vi "Autonomous Independent.vi"() -> ()   [LabVIEW 2020]
doc: "This VI is called when autonomous begins, and will automatically be terminated when autonomous ends. You can carry out timed or sensor driven robot movement independently without needing to return to the caller."
uses:
  <vilib>/Rock Robotics/WPI/ThirdParty/REV Robotics/REVLib/Typedef/Spark MAX Sensor Type.ctl
  <vilib>/Rock Robotics/WPI/Solenoid/WPI_SolenoidValue.ctl
  <vilib>/Rock Robotics/WPI/Utilities/WPI_GetSetVariantRefNum.vi
  <vilib>/Rock Robotics/Network Tables/NT Read String.vi
  <vilib>/Rock Robotics/Network Tables/NT Write Numeric Array.vi
  <vilib>/Rock Robotics/Network Tables/NT Write Number.vi
  Robot Global Data.vi
  <vilib>/Rock Robotics/WPI/Solenoid/WPI_SolenoidSetEnum.vi
  <vilib>/Rock Robotics/WPI/RobotDrive/WPI_RobotDriveArcadeDrive_Standard(NoSaturation).vi
panel:
  out "Right Drive Encoder 2":dbl format="%#.3f"
  out "Sensor Position 2":dbl
  out "Timestamp 2":u32
  out "Sensor Position":dbl
  out "Timestamp":u32
  in  "error in 2":errorcluster
  out "Real Yaw":dbl
  out "Right Drive Encoder":dbl format="%#.3f"
  in  "error in":errorcluster
  # "Be sure to right-click and choose Data Operations>>Make Current Value default if you want to save the array values with the VI"
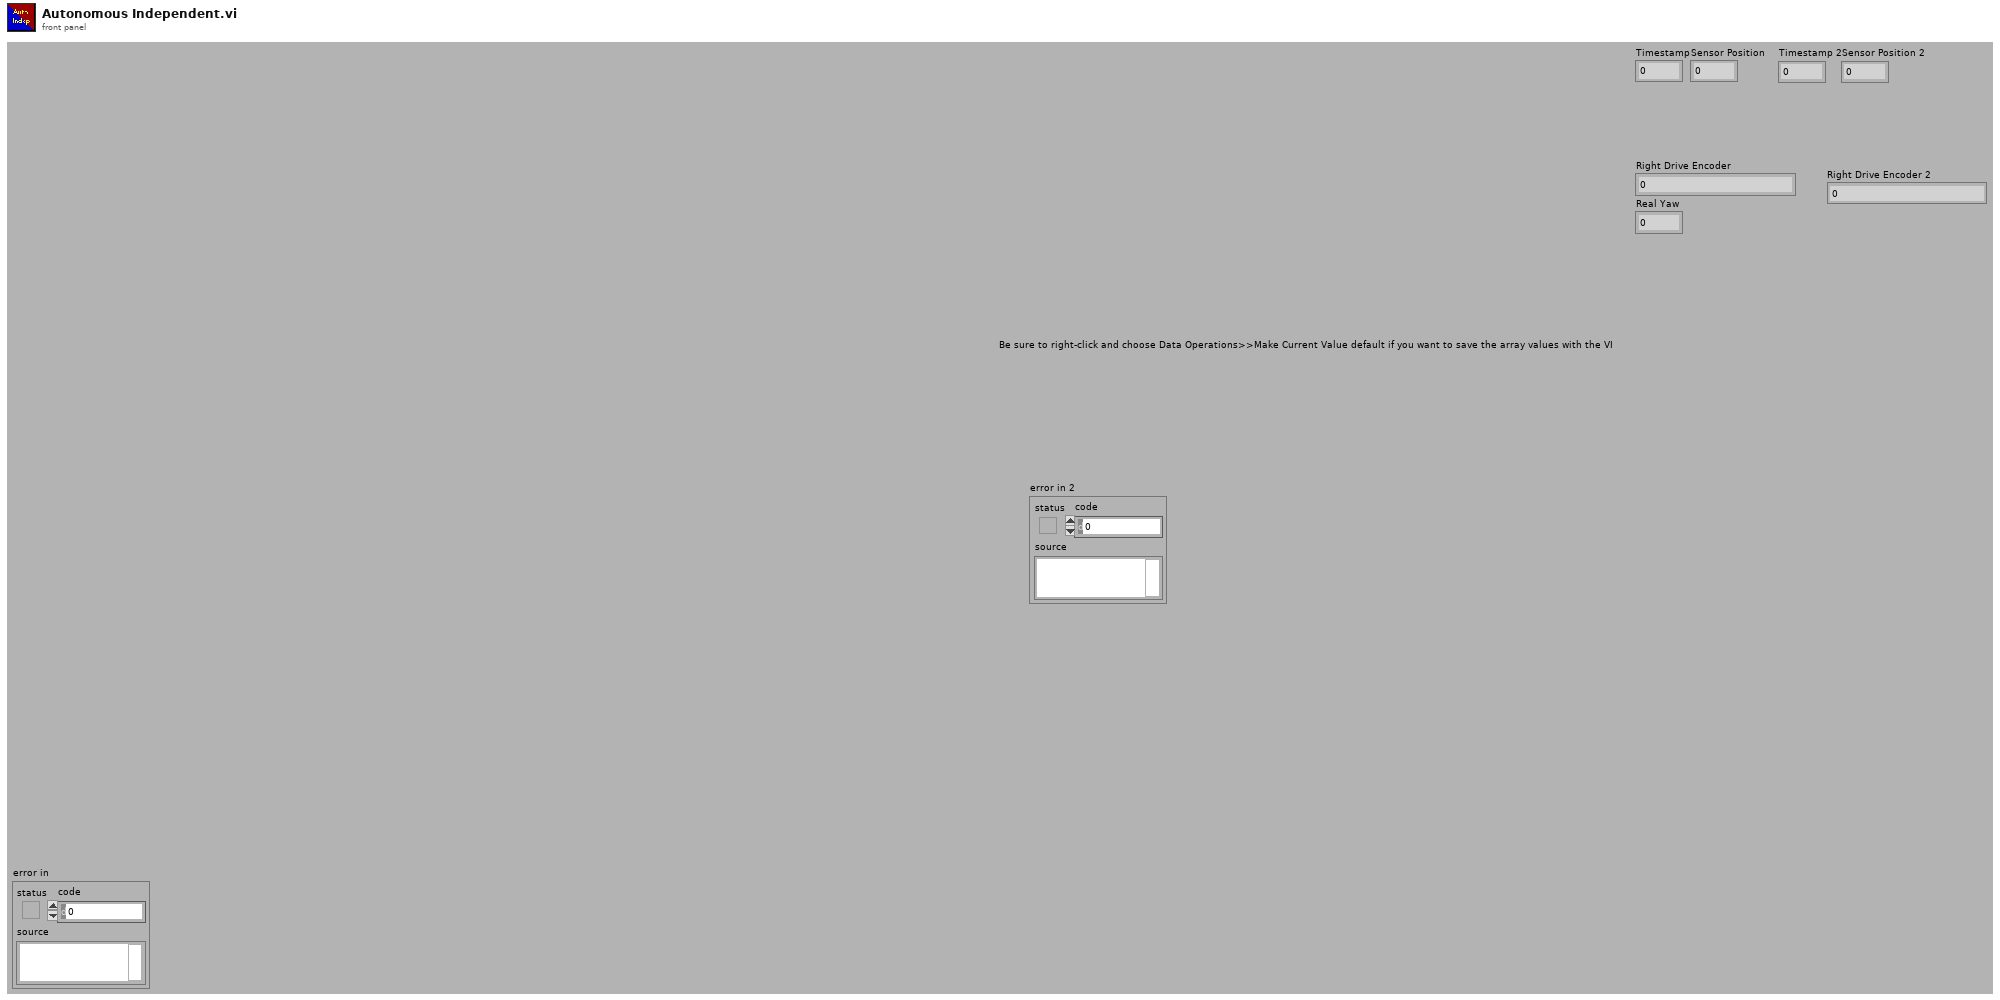
[diagram p1: front panel]
types:
  T1 = typedef "Spark MAX Sensor Type.ctl" = enum16{"No Sensor", "Hall Sensor", "Encoder", "-Not Available-", "Analog", "Alternate Encoder", "Duty Cycle"}
  T2 = typedef "WPI_JoystickDevRef.ctl" = cluster{"Device":T3}
  T3 = typedef "WPI_JoystickDeviceEnum.ctl" = enum16{"USB 0", "USB 1", "USB 2", "USB 3", "USB 4", "USB 5"}
  T4 = typedef "WPI_RobotDriveDevRef.ctl" = cluster{"DevStatus":errorcluster, "Motors[]":T5[], "Square Inputs":bool, "Max Output":dbl}
  T5 = typedef "WPI_MotorControlDeviceRef.ctl" = cluster{"DeviceStatus":errorcluster, "Type":T6, "PWM":cluster{"PWM Channel":T7, "DeadBand":T8}, "CAN":cluster{"Device Number":u8, "SetOutput VI Ref":variant, "GetOutput VI Ref":variant, "Enable VI Ref":variant, "Disable VI Ref":variant, "Data":variant}, "Invert":bool, "DIO PWM":cluster{"PWM \"Enable\" Channel":T7, "DIOChannel":T9, "PWM Rate":dbl}}
  T6 = typedef "WPI_MotorControlType.ctl" = enum16{"PWM", "CAN", "DIO PWM"}
  T7 = typedef "FPGA_DIOPWMChannel.ctl" = enum8{"PWM 0", "PWM 1", "PWM 2", "PWM 3", "PWM 4", "PWM 5", "PWM 6", "PWM 7", "PWM 8", "PWM 9", "PWM MXP 0", "PWM MXP 1", "PWM MXP 2", "PWM MXP 3", "PWM MXP 4", "PWM MXP 5", "PWM MXP 6", "PWM MXP 7", "PWM MXP 8", "PWM MXP 9", "Invalid"}
  T8 = typedef "WPI_PWMDeadband.ctl" = cluster{"Name":string, "maxPositivePwm":i32, "minPositivePwm":i32, "centerPwm":i32, "maxNegativePwm":i32, "minNegativePwm":i32, "angularRange":u16}
  T9 = typedef "FPGA_DIOChannel.ctl" = enum8{"DIO 0", "DIO 1", "DIO 2", "DIO 3", "DIO 4", "DIO 5", "DIO 6", "DIO 7", "DIO 8", "DIO 9", "DIO MXP 0", "DIO MXP 1", "DIO MXP 2", "DIO MXP 3", "DIO MXP 4", "DIO MXP 5", "DIO MXP 6", "DIO MXP 7", "DIO MXP 8", "DIO MXP 9", "DIO MXP 10", "DIO MXP 11", "DIO MXP 12", "DIO MXP 13", "DIO MXP 14", "DIO MXP 15", "SPI Port CS1", "SPI Port CS2", "SPI Port CS3", "SPI Port MISO", "SPI Port MOSI", "Invalid"}
  T10 = cluster{"Motors[][0]":T5, "Motors[][1]":T5, "Motors[][2]":T5, "Motors[][3]":T5, "Motors[][4]":T5, "Motors[][5]":T5, "Motors[][6]":T5, "Motors[][7]":T5, "Motors[][8]":T5}
  T11 = typedef "WPI_SolenoidValue.ctl" = enum16{"Off", "On", "Forward", "Reverse"}
  T12 = typedef "WPI_SolenoidDevRef.ctl" = cluster{"DevStatus":errorcluster, "Pneumatics Control Module":u8, "Forward Solenoid Channel":T13, "Reverse Solenoid Channel":T13}
  T13 = typedef "WPI_SolenoidChannel.ctl" = enum8{"Solenoid 0", "Solenoid 1", "Solenoid 2", "Solenoid 3", "Solenoid 4", "Solenoid 5", "Solenoid 6", "Solenoid 7", "Solenoid 8", "Solenoid 9", "Solenoid 10", "Solenoid 11", "Solenoid 12", "Solenoid 13", "Solenoid 14", "Solenoid 15", "Invalid"}
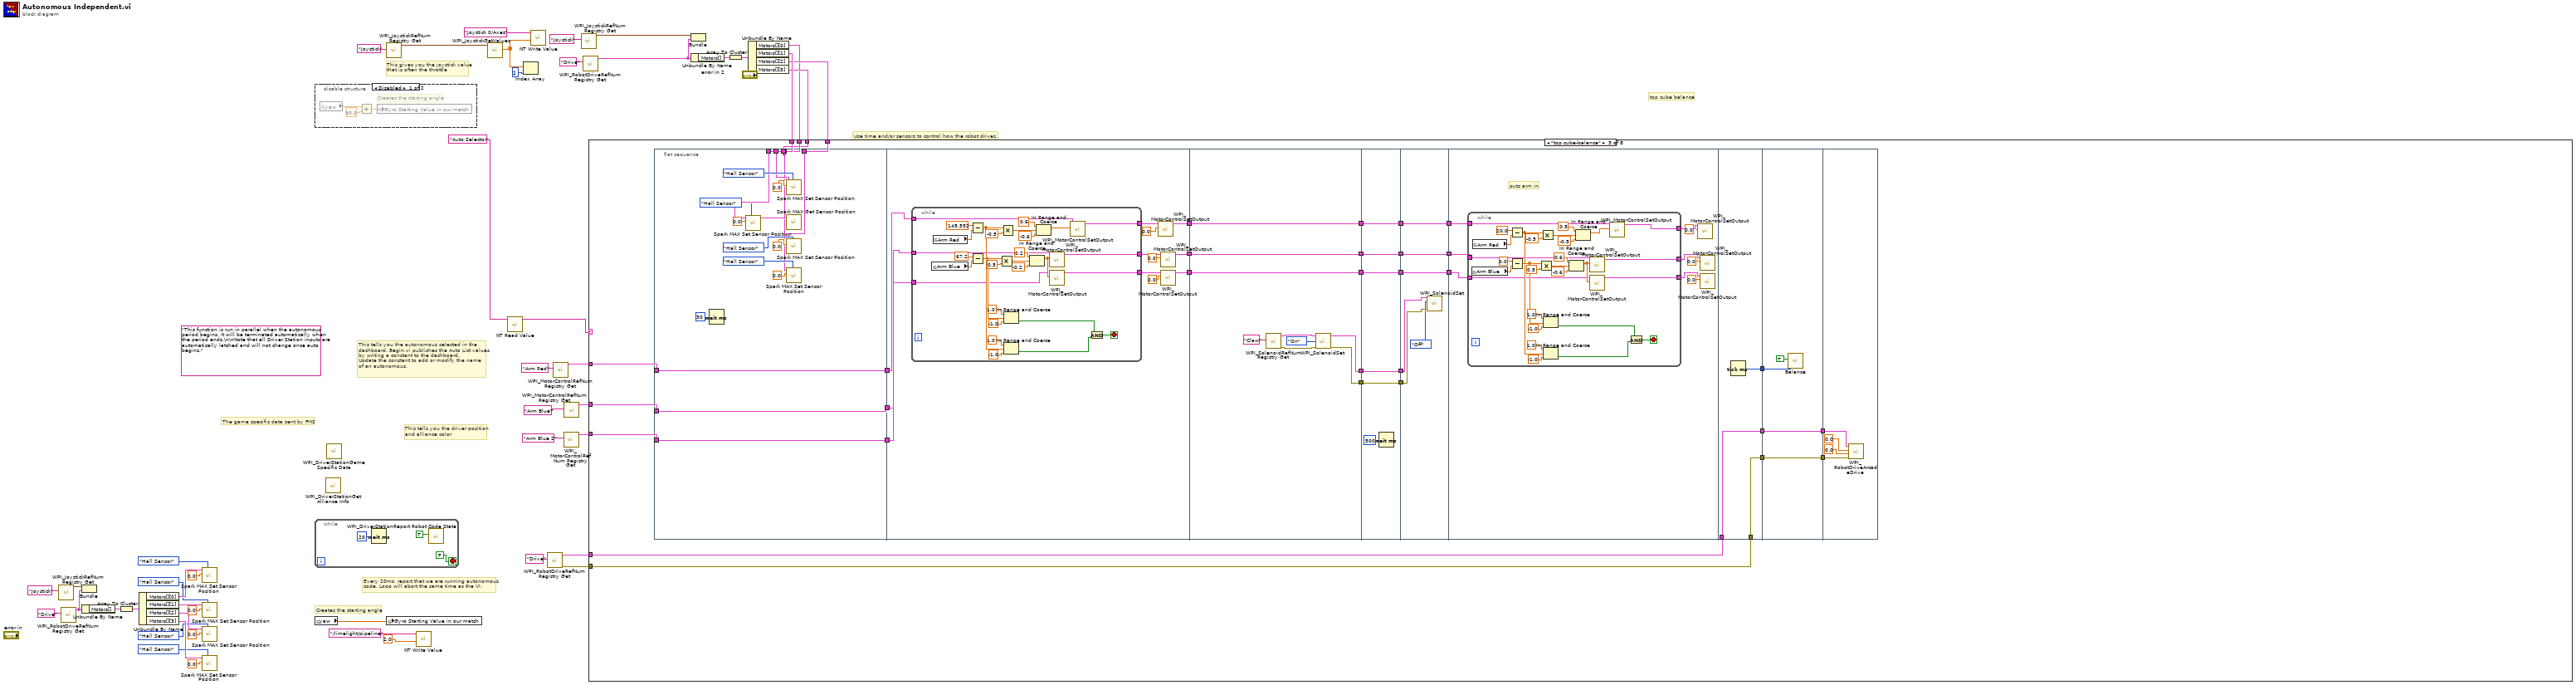
[diagram p0: block diagram]
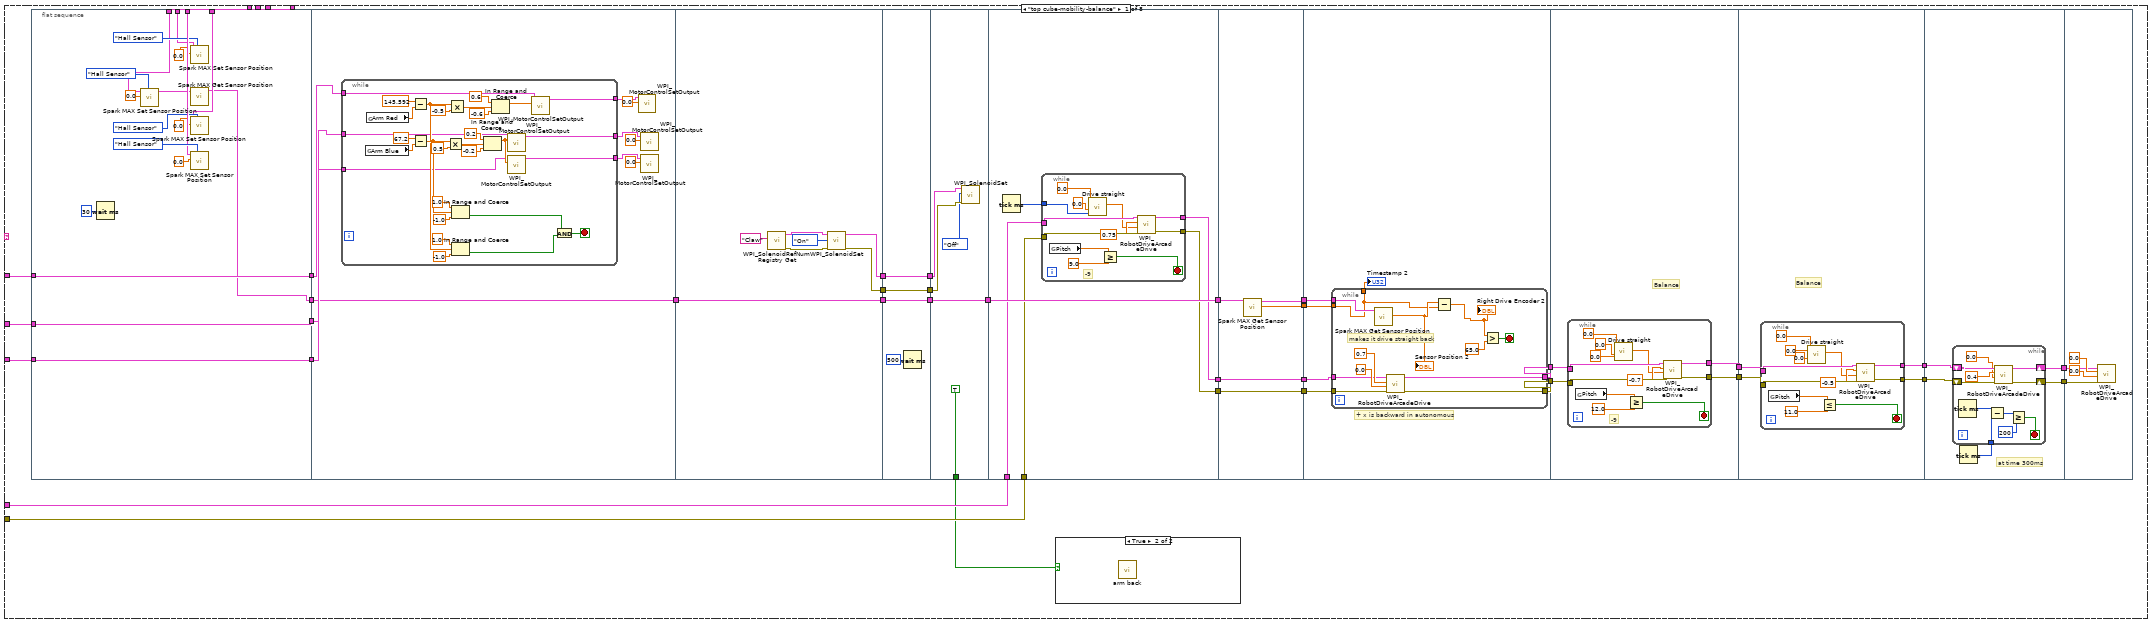
[diagram p3: hidden frame]
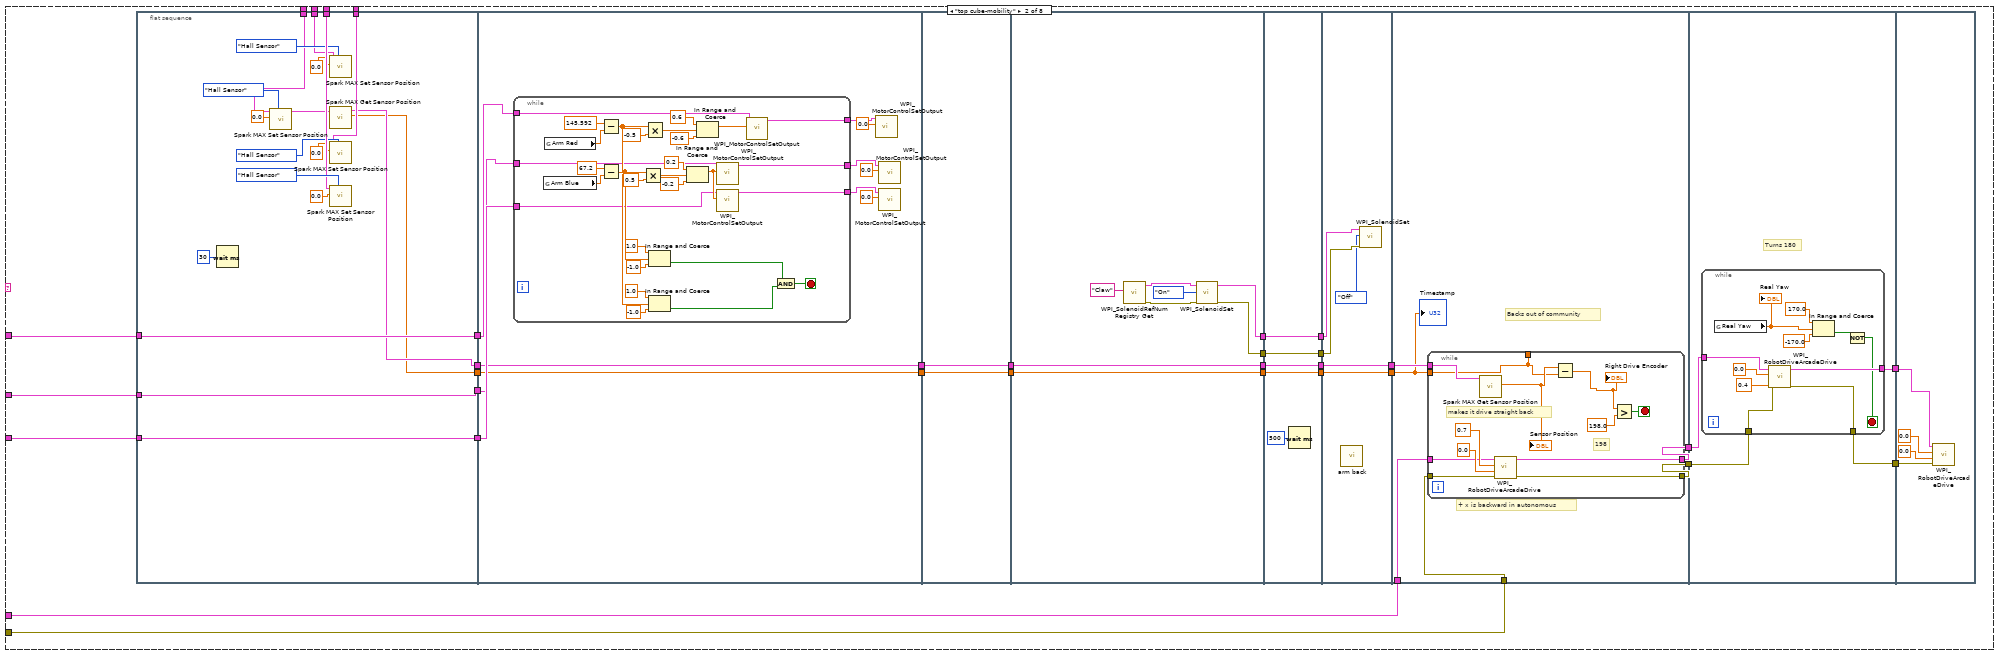
[diagram p5: hidden frame]
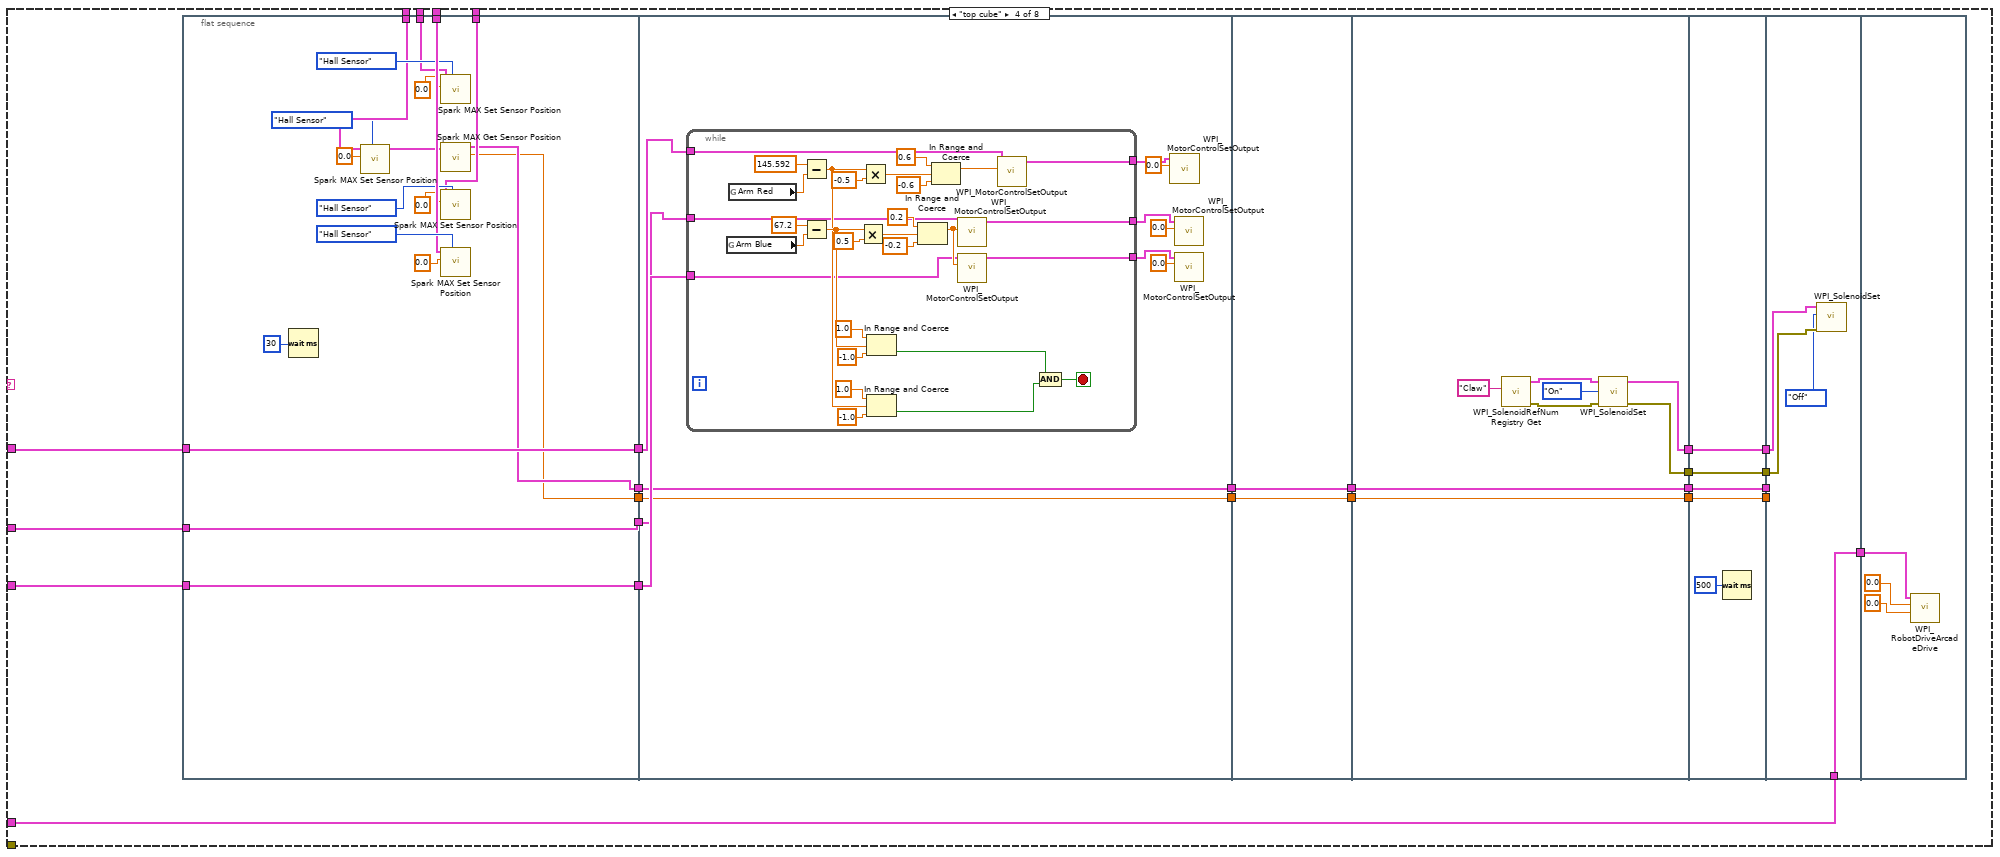
[diagram p6: hidden frame]
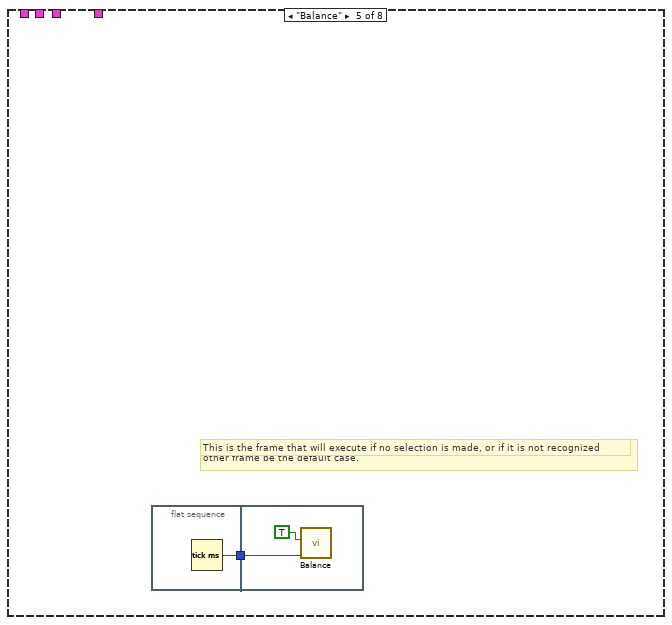
[diagram p7: hidden frame]
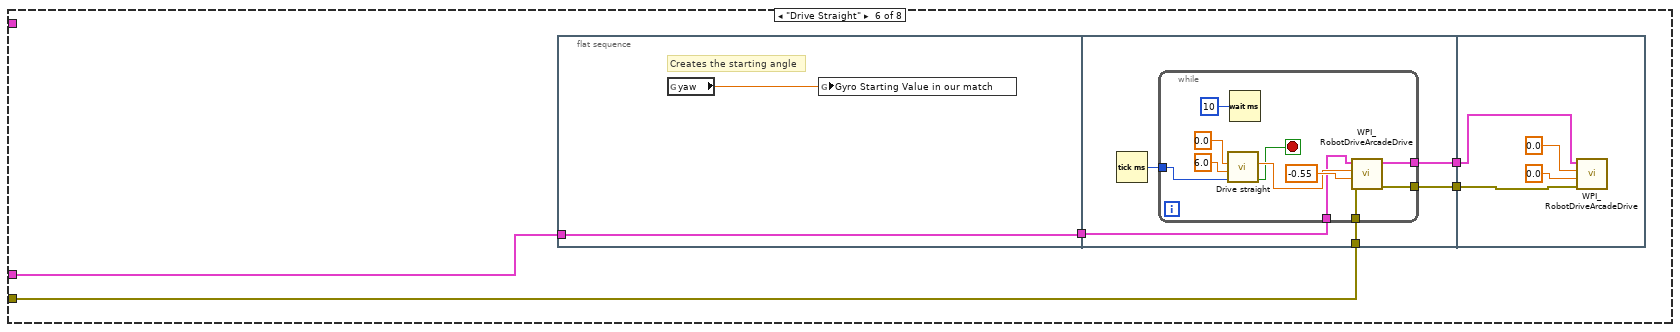
[diagram p8: hidden frame]
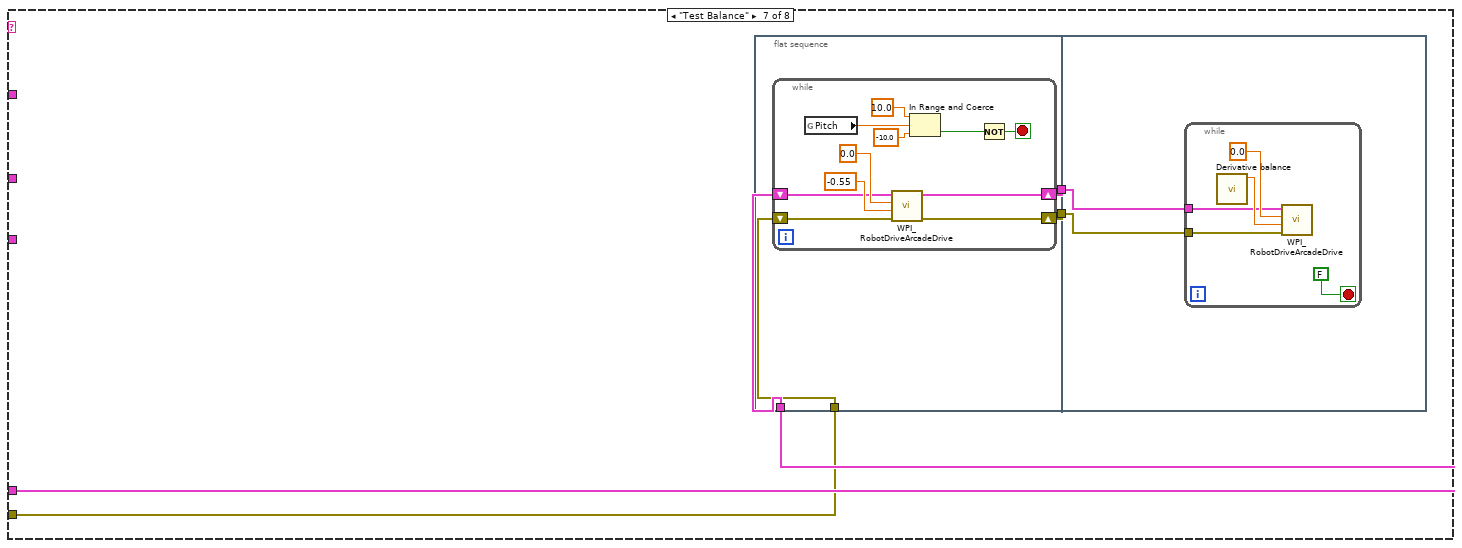
[diagram p9: hidden frame]
diagram:
  (unwired) "This function is run in parallel when the autonomous period begins. It will be terminated automatically when the period ends.\n\nNote that all Driver Station inputs are automatically latched and will not change once auto begins."
  # "top cube balance"
  # "Creates the starting angle"
  # "The game specific data sent by FMS"
  # "This tells you the autonomous selected in the \ndashboard. Begin.vi publishes the Auto List values\nby writing a constant to the dashboard.\nUpdate the constant to add or modify the name\nof an autonomous."
  # "Every 20ms, report that we are running autonomous\ncode. Loop will abort the same time as the VI."
  # "This gives you the joystick value\nthat is often the throttle"
  # "Use time and/or sensors to control how the robot drives."
  # "This tells you the driver position\nand alliance color"
  n1 = call <vilib>:"WPI_JoystickRefNum Registry Get.vi"("refnum name"="Joystick") -> ("JoystickDevRef"=w26:T2)  [unwired: 1 in, 9 out]
  n2 = call <vilib>:"WPI_RobotDriveRefNum Registry Get.vi"("refnum name"="Drive") -> ("RobotDriveDevRef"=w22:T4)  [unwired: 1 in, 9 out]
  n3 = Bundle("JoystickDevRef"=w26, "RobotDriveDevRef"=w22) -> ()  [unwired: 2 out]
  n4 = Unbundle By Name(w22) -> ("Motors[]"=w25:T5[])
  n5 = Array To Cluster(array=w25) -> (cluster=w24:T10)
  n6 = Unbundle By Name(w24) -> ("Motors[][0]"=w21:T5, "Motors[][1]"=w20:T5, "Motors[][2]"=w19:T5, "Motors[][3]"=w18:T5)
  n7 = call <vilib>:"Spark MAX Set Sensor Position.vi"("Sensor Type (Hall Sensor)"=Spark_MAX_Sensor_Type."Hall Sensor", "Position"=0.0, "MotorControlDeviceRef"=w21) -> ()  [unwired: 7 in, 2 out]
  n8 = call <vilib>:"Spark MAX Set Sensor Position.vi"("Sensor Type (Hall Sensor)"=Spark_MAX_Sensor_Type."Hall Sensor", "Position"=0.0, "MotorControlDeviceRef"=w20) -> ()  [unwired: 7 in, 2 out]
  n9 = call <vilib>:"Spark MAX Set Sensor Position.vi"("Sensor Type (Hall Sensor)"=Spark_MAX_Sensor_Type."Hall Sensor", "Position"=0.0, "MotorControlDeviceRef"=w19) -> ()  [unwired: 7 in, 2 out]
  n10 = call <vilib>:"Spark MAX Set Sensor Position.vi"("Sensor Type (Hall Sensor)"=Spark_MAX_Sensor_Type."Hall Sensor", "Position"=0.0, "MotorControlDeviceRef"=w18) -> ()  [unwired: 7 in, 2 out]
  n11 = disable-structure shown="Disabled" {
    frame Disabled {
      # "Creates the starting angle"
      n12 = global read "Robot Global Data.vi" "yaw"() -> (w49:dbl)
      n13 = Add(x=w49, y=90.0) -> (x+y=w50:dbl)
      n14 = global write "Robot Global Data.vi" "Gyro Starting Value in our match"(w50) -> ()
    }
    frame Enabled {
    }
  }
  n15 = while {
    stop <- FALSE stop-if-true
    n16 = Wait (ms)(milliseconds to wait=u32 20) -> ()  [unwired: 1 out]
    n17 = call <vilib>:"WPI_DriverStationReport Robot Code State.vi"("Autonomous"=TRUE) -> ()  [unwired: 10 in, 1 out]
  }
  n18 = global read "Robot Global Data.vi" "yaw"() -> (w40:dbl)
  n19 = call <vilib>:"WPI_DriverStationGet Alliance Info.vi"() -> ()  [unwired: 12 out]
  n20 = call <vilib>:"WPI_DriverStationGame Specific Data.vi"() -> ()  [unwired: 11 in, 1 out]
  n21 = call <vilib>:"WPI_JoystickRefNum Registry Get.vi"("refnum name"="Joystick") -> ("JoystickDevRef"=w46:T2)  [unwired: 1 in, 9 out]
  n22 = global write "Robot Global Data.vi" "Gyro Starting Value in our match"(w40) -> ()
  n23 = call-poly <vilib>:"NT Write Value.vi"("value"=2.0, "name"="/limelight/pipeline" ("Name")) -> ()  [unwired: 9 in, 1 out]
  n24 = call <vilib>:"WPI_JoystickGetValues.vi"("JoystickDevRef"=w46) -> ("Axes"=w42:dbl[])  [unwired: 6 in, 4 out]
  n25 = call-poly <vilib>:"NT Read Value.vi"("name"="Auto Selector" ("Name")) -> ("value"=w43:string)  [unwired: 8 in, 2 out]
  n26 = Index Array(array=w42, index=2) -> ()  [unwired: 1 out]
  n27 = call-poly <vilib>:"NT Write Value.vi"("value"=w42, "name"="Joystick 0/Axes" ("Name")) -> ()  [unwired: 9 in, 1 out]
  n28 = call <vilib>:"WPI_RobotDriveRefNum Registry Get.vi"("refnum name"="Drive") -> ("error out"=w29:errorcluster, "RobotDriveDevRef"=w30:T4)  [unwired: 9 in]
  n29 = call <vilib>:"WPI_MotorControlRefNum Registry Get.vi"("refnum name"="Arm Red") -> ("MotorControlDevRef"=w34:T5)  [unwired: 9 in, 1 out]
  n30 = call <vilib>:"WPI_MotorControlRefNum Registry Get.vi"("refnum name"="Arm Blue 2") -> ("MotorControlDevRef"=w32:T5)  [unwired: 9 in, 1 out]
  n31 = call <vilib>:"WPI_MotorControlRefNum Registry Get.vi"("refnum name"="Arm Blue") -> ("MotorControlDevRef"=w33:T5)  [unwired: 9 in, 1 out]
  n32 = call <vilib>:"WPI_JoystickRefNum Registry Get.vi"("refnum name"="Joystick") -> ("JoystickDevRef"=w7:T2)  [unwired: 1 in, 9 out]
  n33 = call <vilib>:"WPI_RobotDriveRefNum Registry Get.vi"("refnum name"="Drive") -> ("RobotDriveDevRef"=w10:T4)  [unwired: 1 in, 9 out]
  n34 = Bundle("JoystickDevRef"=w7, "RobotDriveDevRef"=w10) -> ()  [unwired: 2 out]
  n35 = Unbundle By Name(w10) -> ("Motors[]"=w8:T5[])
  n36 = Array To Cluster(array=w8) -> (cluster=w9:T10)
  n37 = Unbundle By Name(w9) -> ("Motors[][0]"=w1:T5, "Motors[][1]"=w4:T5, "Motors[][2]"=w2:T5, "Motors[][3]"=w3:T5)
  n38 = case shown="\"top cube-balance\"" w43 {
    tunnel: w34 -> [w90 w289 w431 w592 _ _ _ _]
    tunnel: w33 -> [w89 w288 w430 w591 _ _ _ _]
    tunnel: w32 -> [w88 w287 w429 w590 _ _ _ _]
    tunnel: w30 -> [w72 w282 w428 w567 _ w679 w708 _]
    tunnel: w29 -> [w71 w281 w427 _ _ w678 w707 _]
    tunnel: w4 -> [w77 w267 w425 w577 _ _ _ _]
    tunnel: w3 -> [w76 w266 w423 w576 _ _ _ _]
    tunnel: w2 -> [w75 w265 w422 w575 _ _ _ _]
    tunnel: w1 -> [w74 w264 w424 w574 _ _ _ _]
    frame "top cube-mobility-balance" {
      n39 = flat-sequence {
        tunnel: w88 -> [w108]
        tunnel: w89 -> [w107]
        tunnel: w90 -> [w106]
        tunnel: [w108] -> w83
        tunnel: [w96] -> w80
        tunnel: [w107] -> w79
        tunnel: [w106] -> w78
        tunnel: w77 -> [w94]
        tunnel: w76 -> [w103]
        tunnel: w75 -> [w100]
        tunnel: w74 -> [w97]
        tunnel: w83 -> [w118]
        tunnel: [w117] -> w55
        tunnel: w80 -> [w117]
        tunnel: w79 -> [w115]
        tunnel: w78 -> [w116]
        tunnel: [w154] -> w87
        tunnel: [w153] -> w85
        tunnel: [w152] -> w81
        tunnel: w55 -> [w152]
        tunnel: w87 -> [w158]
        tunnel: [w158] -> w86
        tunnel: w85 -> [w157]
        tunnel: [w157] -> w84
        tunnel: [w156] -> w82
        tunnel: w81 -> [w156]
        tunnel: w86 -> [w163]
        tunnel: w84 -> [w162]
        tunnel: [w161] -> w73
        tunnel: w82 -> [w161]
        tunnel: [TRUE] -> w54
        tunnel: w73 -> [w169]
        tunnel: [w169] -> w68
        tunnel: w72 -> [w167]
        tunnel: w71 -> [w166]
        tunnel: [w165] -> w66
        tunnel: [w164] -> w64
        tunnel: w68 -> [w184]
        tunnel: [w183] -> w67
        tunnel: w66 -> [w186]
        tunnel: [w186] -> w65
        tunnel: w64 -> [w185]
        tunnel: [w185] -> w63
        tunnel: [w182] -> w62
        tunnel: [w193] -> w70
        tunnel: [w192] -> w69
        tunnel: w67 -> [w191]
        tunnel: w65 -> [w190]
        tunnel: w63 -> [w189]
        tunnel: w62 -> [w188]
        tunnel: w70 -> [w209]
        tunnel: [w207] -> w61
        tunnel: w69 -> [w208]
        tunnel: [w206] -> w60
        tunnel: w61 -> [w225]
        tunnel: w60 -> [w224]
        tunnel: [w223] -> w59
        tunnel: [w222] -> w58
        tunnel: w59 -> [w241]
        tunnel: w58 -> [w240]
        tunnel: [w239] -> w57
        tunnel: [w238] -> w56
        tunnel: w57 -> [w255]
        tunnel: w56 -> [w254]
        frame #0 {
          n40 = Wait (ms)(milliseconds to wait=u32 30) -> ()  [unwired: 1 out]
          n41 = call <vilib>:"Spark MAX Set Sensor Position.vi"("Sensor Type (Hall Sensor)"=Spark_MAX_Sensor_Type."Hall Sensor", "Position"=0.0, "MotorControlDeviceRef"=w94) -> ("MotorControlDeviceRef"=w93:T5)  [unwired: 7 in, 1 out]
          n42 = call <vilib>:"Spark MAX Set Sensor Position.vi"("Sensor Type (Hall Sensor)"=Spark_MAX_Sensor_Type."Hall Sensor", "Position"=0.0, "MotorControlDeviceRef"=w97) -> ()  [unwired: 7 in, 2 out]
          n43 = call <vilib>:"Spark MAX Get Sensor Position.vi"("MotorControlDevRef in"=w93) -> ("MotorControlDevRef out"=w96:T5)  [unwired: 7 in, 3 out]
          n44 = call <vilib>:"Spark MAX Set Sensor Position.vi"("Sensor Type (Hall Sensor)"=Spark_MAX_Sensor_Type."Hall Sensor", "Position"=0.0, "MotorControlDeviceRef"=w100) -> ()  [unwired: 7 in, 2 out]
          n45 = call <vilib>:"Spark MAX Set Sensor Position.vi"("Sensor Type (Hall Sensor)"=Spark_MAX_Sensor_Type."Hall Sensor", "Position"=0.0, "MotorControlDeviceRef"=w103) -> ()  [unwired: 7 in, 2 out]
        }
        frame #1 {
          n46 = while {
            tunnel: w116 -> [w124]
            tunnel: w115 -> [w123]
            tunnel: w118 -> [w122]
            tunnel: [w119] -> w114
            tunnel: [w121] -> w113
            tunnel: [w120] -> w112
            stop <- w147 stop-if-true
            n47 = global read "Robot Global Data.vi" "Arm Blue"() -> (w127:dbl)
            n48 = global read "Robot Global Data.vi" "Arm Red"() -> (w138:dbl)
            n49 = Subtract(x=145.592, y=w138) -> (x-y=w125:dbl)
            n50 = Subtract(x=67.2, y=w127) -> (x-y=w126:dbl)
            n51 = Multiply(x=w126, y=0.5) -> (x*y=w135:dbl)
            n52 = Multiply(x=w125, y=-0.5) -> (x*y=w134:dbl)
            n53 = In Range and Coerce(upper limit=1.0, x=w126, lower limit=-1.0) -> (In Range?=w146:bool)  [unwired: 1 out]
            n54 = In Range and Coerce(upper limit=1.0, x=w125, lower limit=-1.0) -> (In Range?=w145:bool)  [unwired: 1 out]
            n55 = In Range and Coerce(upper limit=0.2, x=w135, lower limit=-0.2) -> (coerced(x)=w130:dbl)  [unwired: 1 out]
            n56 = In Range and Coerce(upper limit=0.6, x=w134, lower limit=-0.6) -> (coerced(x)=w131:dbl)  [unwired: 1 out]
            n57 = call <vilib>:"WPI_MotorControlSetOutput.vi"("Output"=w130, "MotorControlDevRef"=w123) -> ("MotorControlDevRef"=w119:T5)  [unwired: 7 in, 2 out]
            n58 = call <vilib>:"WPI_MotorControlSetOutput.vi"("Output"=w130, "MotorControlDevRef"=w122) -> ("MotorControlDevRef"=w121:T5)  [unwired: 7 in, 2 out]
            n59 = call <vilib>:"WPI_MotorControlSetOutput.vi"("Output"=w131, "MotorControlDevRef"=w124) -> ("MotorControlDevRef"=w120:T5)  [unwired: 7 in, 2 out]
            n60 = And(x=w146, y=w145) -> (x .and. y?=w147:bool)
          }
          n61 = call <vilib>:"WPI_MotorControlSetOutput.vi"("Output"=0.0, "MotorControlDevRef"=w112) -> ()  [unwired: 7 in, 3 out]
          n62 = call <vilib>:"WPI_MotorControlSetOutput.vi"("Output"=0.0, "MotorControlDevRef"=w114) -> ()  [unwired: 7 in, 3 out]
          n63 = call <vilib>:"WPI_MotorControlSetOutput.vi"("Output"=0.0, "MotorControlDevRef"=w113) -> ()  [unwired: 7 in, 3 out]
        }
        frame #2 {
          n64 = call <vilib>:"WPI_SolenoidRefNum Registry Get.vi"("refnum name"="Claw") -> ("error out"=w151:errorcluster, "SolenoidDevRef"=w150:T12)  [unwired: 9 in]
          n65 = call-poly <vilib>:"WPI_SolenoidSet.vi"("error in (no error)"=w151, "Value"=WPI_SolenoidValue."On", "SolenoidDevRef"=w150) -> ("error out"=w153:errorcluster, "SolenoidDevRef"=w154:T12)  [unwired: 7 in]
        }
        frame #3 {
          n66 = Wait (ms)(milliseconds to wait=u32 500) -> ()  [unwired: 1 out]
        }
        frame #4 {
          n67 = call-poly <vilib>:"WPI_SolenoidSet.vi"("error in (no error)"=w162, "Value"=WPI_SolenoidValue."Off", "SolenoidDevRef"=w163) -> ()  [unwired: 7 in, 2 out]
        }
        frame #5 {
          n68 = Tick Count (ms)() -> (millisecond timer value=w168:u32)
          n69 = while {
            tunnel: [w179] -> w165
            tunnel: w167 -> [w178]
            tunnel: w166 -> [w177]
            tunnel: [w175] -> w164
            tunnel: w168 -> [w171]
            stop <- w181 stop-if-true
            # "-9"
            n70 = global read "Robot Global Data.vi" "Pitch"() -> (w176:dbl)
            n71 = call "Drive straight.vi"("Start Time"=w171, "Length(seconds)"=0.0, "Desired angle"=0.0) -> ("X Power"=w172:dbl)  [unwired: 7 in, 1 out]
            n72 = Greater Or Equal?(x=w176, y=9.0) -> (x >= y?=w181:bool)
            n73 = call-poly <vilib>:"WPI_RobotDriveArcadeDrive.vi"("error in (no error)"=w177, "Y axis value"=w172, "X axis value"=0.75 ("Y axis value"), "RobotDriveDevRef"=w178) -> ("error out"=w175:errorcluster, "RobotDriveDevRef"=w179:T4)  [unwired: 5 in, 1 out]
          }
        }
        frame #6 {
          n74 = call <vilib>:"Spark MAX Get Sensor Position.vi"("MotorControlDevRef in"=w184) -> ("Sensor Position"=w182:dbl, "MotorControlDevRef out"=w183:T5)  [unwired: 7 in, 2 out]
        }
        frame #7 {
          # "+ x is backward in autonomous"
          n75 = while {
            tunnel: [w203] -> w193
            tunnel: [w202] -> w192
            tunnel: w190 -> [w200]
            tunnel: w191 -> [w198]
            tunnel: w189 -> [w195]
            tunnel: w188 -> [w194]
            tunnel: [w194] -> w187
            stop <- w201 stop-if-true
            # "makes it drive straight back"
            n76 = call <vilib>:"Spark MAX Get Sensor Position.vi"("MotorControlDevRef in"=w198) -> ("Sensor Position"=w196:dbl)  [unwired: 7 in, 3 out]
            "Sensor Position 2" <- w196
            n77 = call-poly <vilib>:"WPI_RobotDriveArcadeDrive.vi"("error in (no error)"=w195, "Y axis value"=0.0, "X axis value"=0.7, "RobotDriveDevRef"=w200) -> ("error out"=w202:errorcluster, "RobotDriveDevRef"=w203:T4)  [unwired: 5 in, 1 out]
            n78 = Subtract(x=w196, y=w194) -> (x-y=w197:dbl)
            "Right Drive Encoder 2" <- w197
            n79 = Greater?(x=w197, y=65.0) -> (0:w201:bool)
          }
          "Timestamp 2" <- w187
        }
        frame #8 {
          # "Balance"
          n80 = while {
            tunnel: [w219] -> w207
            tunnel: w209 -> [w218]
            tunnel: w208 -> [w217]
            tunnel: [w215] -> w206
            stop <- w221 stop-if-true
            # "-9"
            n81 = global read "Robot Global Data.vi" "Pitch"() -> (w216:dbl)
            n82 = call "Drive straight.vi"("Start Time"=0.0, "Length(seconds)"=0.0, "Desired angle"=0.0) -> ("X Power"=w212:dbl)  [unwired: 7 in, 1 out]
            n83 = Greater Or Equal?(x=w216, y=12.0) -> (x >= y?=w221:bool)
            n84 = call-poly <vilib>:"WPI_RobotDriveArcadeDrive.vi"("error in (no error)"=w217, "Y axis value"=w212, "X axis value"=-0.7 ("Y axis value"), "RobotDriveDevRef"=w218) -> ("error out"=w215:errorcluster, "RobotDriveDevRef"=w219:T4)  [unwired: 5 in, 1 out]
          }
        }
        frame #9 {
          # "Balance"
          n85 = while {
            tunnel: [w235] -> w223
            tunnel: w225 -> [w234]
            tunnel: w224 -> [w233]
            tunnel: [w231] -> w222
            stop <- w237 stop-if-true
            n86 = global read "Robot Global Data.vi" "Pitch"() -> (w232:dbl)
            n87 = call "Drive straight.vi"("Start Time"=0.0, "Length(seconds)"=0.0, "Desired angle"=0.0) -> ("X Power"=w227:dbl)  [unwired: 7 in, 1 out]
            n88 = Less Or Equal?(x=w232, y=11.0) -> (x <= y?=w237:bool)
            n89 = call-poly <vilib>:"WPI_RobotDriveArcadeDrive.vi"("error in (no error)"=w233, "Y axis value"=w227, "X axis value"=-0.5 ("Y axis value"), "RobotDriveDevRef"=w234) -> ("error out"=w231:errorcluster, "RobotDriveDevRef"=w235:T4)  [unwired: 5 in, 1 out]
          }
        }
        frame #10 {
          # "at time 300ms"
          n90 = Tick Count (ms)() -> (millisecond timer value=w242:u32)
          n91 = while {
            shift-right: [w251] -> w239
            shift-left: w241 -> [w253]
            shift-right: [w250] -> w238
            shift-left: w240 -> [w252]
            tunnel: w242 -> [w248]
            stop <- w245 stop-if-true
            n92 = Tick Count (ms)() -> (millisecond timer value=w249:u32)
            n93 = Subtract(x=w249, y=w248) -> (x-y=w247:u32)
            n94 = call-poly <vilib>:"WPI_RobotDriveArcadeDrive.vi"("error in (no error)"=w252, "Y axis value"=0.0 ("X axis value"), "X axis value"=0.4 ("Y axis value"), "RobotDriveDevRef"=w253) -> ("error out"=w250:errorcluster, "RobotDriveDevRef"=w251:T4)  [unwired: 5 in, 1 out]
            n95 = Greater Or Equal?(x=w247, y=u32 200) -> (x >= y?=w245:bool)
          }
        }
        frame #11 {
          n96 = call-poly <vilib>:"WPI_RobotDriveArcadeDrive.vi"("error in (no error)"=w254, "Y axis value"=0.0, "X axis value"=0.0, "RobotDriveDevRef"=w255) -> ()  [unwired: 5 in, 3 out]
        }
      }
      n97 = case shown="True" w54 {
        frame False {
        }
        frame True {
          n98 = call "arm back.vi"() -> ()  [unwired: 12 in]
        }
      }
    }
    frame "top cube-mobility" {
      n99 = flat-sequence {
        tunnel: w287 -> [w308]
        tunnel: w288 -> [w307]
        tunnel: w289 -> [w306]
        tunnel: [w308] -> w276
        tunnel: [w296] -> w270
        tunnel: [w307] -> w269
        tunnel: [w306] -> w268
        tunnel: w267 -> [w293]
        tunnel: w266 -> [w303]
        tunnel: w265 -> [w300]
        tunnel: w264 -> [w297]
        tunnel: [w295] -> w258
        tunnel: w276 -> [w319]
        tunnel: [w318] -> w271
        tunnel: w270 -> [w318]
        tunnel: w269 -> [w316]
        tunnel: w268 -> [w317]
        tunnel: [w315] -> w259
        tunnel: w258 -> [w315]
        tunnel: [w350] -> w272
        tunnel: w271 -> [w350]
        tunnel: [w349] -> w260
        tunnel: w259 -> [w349]
        tunnel: [w358] -> w286
        tunnel: [w357] -> w284
        tunnel: [w356] -> w273
        tunnel: w272 -> [w356]
        tunnel: [w355] -> w261
        tunnel: w260 -> [w355]
        tunnel: w286 -> [w363]
        tunnel: [w363] -> w285
        tunnel: w284 -> [w362]
        tunnel: [w362] -> w283
        tunnel: [w361] -> w274
        tunnel: w273 -> [w361]
        tunnel: [w360] -> w262
        tunnel: w261 -> [w360]
        tunnel: w285 -> [w368]
        tunnel: w283 -> [w367]
        tunnel: [w366] -> w275
        tunnel: w274 -> [w366]
        tunnel: [w365] -> w263
        tunnel: w262 -> [w365]
        tunnel: [w374] -> w280
        tunnel: [w373] -> w279
        tunnel: w282 -> [w372]
        tunnel: w281 -> [w371]
        tunnel: w275 -> [w370]
        tunnel: w263 -> [w369]
        tunnel: w280 -> [w390]
        tunnel: w279 -> [w389]
        tunnel: [w388] -> w278
        tunnel: [w387] -> w277
        tunnel: w278 -> [w403]
        tunnel: w277 -> [w402]
        frame #0 {
          n100 = Wait (ms)(milliseconds to wait=u32 30) -> ()  [unwired: 1 out]
          n101 = call <vilib>:"Spark MAX Set Sensor Position.vi"("Sensor Type (Hall Sensor)"=Spark_MAX_Sensor_Type."Hall Sensor", "Position"=0.0, "MotorControlDeviceRef"=w293) -> ("MotorControlDeviceRef"=w292:T5)  [unwired: 7 in, 1 out]
          n102 = call <vilib>:"Spark MAX Set Sensor Position.vi"("Sensor Type (Hall Sensor)"=Spark_MAX_Sensor_Type."Hall Sensor", "Position"=0.0, "MotorControlDeviceRef"=w297) -> ()  [unwired: 7 in, 2 out]
          n103 = call <vilib>:"Spark MAX Get Sensor Position.vi"("MotorControlDevRef in"=w292) -> ("Sensor Position"=w295:dbl, "MotorControlDevRef out"=w296:T5)  [unwired: 7 in, 2 out]
          n104 = call <vilib>:"Spark MAX Set Sensor Position.vi"("Sensor Type (Hall Sensor)"=Spark_MAX_Sensor_Type."Hall Sensor", "Position"=0.0, "MotorControlDeviceRef"=w300) -> ()  [unwired: 7 in, 2 out]
          n105 = call <vilib>:"Spark MAX Set Sensor Position.vi"("Sensor Type (Hall Sensor)"=Spark_MAX_Sensor_Type."Hall Sensor", "Position"=0.0, "MotorControlDeviceRef"=w303) -> ()  [unwired: 7 in, 2 out]
        }
        frame #1 {
          n106 = while {
            tunnel: w317 -> [w325]
            tunnel: w316 -> [w324]
            tunnel: w319 -> [w323]
            tunnel: [w320] -> w314
            tunnel: [w322] -> w313
            tunnel: [w321] -> w312
            stop <- w348 stop-if-true
            n107 = global read "Robot Global Data.vi" "Arm Blue"() -> (w328:dbl)
            n108 = global read "Robot Global Data.vi" "Arm Red"() -> (w339:dbl)
            n109 = Subtract(x=145.592, y=w339) -> (x-y=w326:dbl)
            n110 = Subtract(x=67.2, y=w328) -> (x-y=w327:dbl)
            n111 = Multiply(x=w327, y=0.5) -> (x*y=w336:dbl)
            n112 = Multiply(x=w326, y=-0.5) -> (x*y=w335:dbl)
            n113 = In Range and Coerce(upper limit=1.0, x=w327, lower limit=-1.0) -> (In Range?=w347:bool)  [unwired: 1 out]
            n114 = In Range and Coerce(upper limit=1.0, x=w326, lower limit=-1.0) -> (In Range?=w346:bool)  [unwired: 1 out]
            n115 = In Range and Coerce(upper limit=0.2, x=w336, lower limit=-0.2) -> (coerced(x)=w331:dbl)  [unwired: 1 out]
            n116 = In Range and Coerce(upper limit=0.6, x=w335, lower limit=-0.6) -> (coerced(x)=w332:dbl)  [unwired: 1 out]
            n117 = call <vilib>:"WPI_MotorControlSetOutput.vi"("Output"=w331, "MotorControlDevRef"=w324) -> ("MotorControlDevRef"=w320:T5)  [unwired: 7 in, 2 out]
            n118 = call <vilib>:"WPI_MotorControlSetOutput.vi"("Output"=w331, "MotorControlDevRef"=w323) -> ("MotorControlDevRef"=w322:T5)  [unwired: 7 in, 2 out]
            n119 = call <vilib>:"WPI_MotorControlSetOutput.vi"("Output"=w332, "MotorControlDevRef"=w325) -> ("MotorControlDevRef"=w321:T5)  [unwired: 7 in, 2 out]
            n120 = And(x=w347, y=w346) -> (x .and. y?=w348:bool)
          }
          n121 = call <vilib>:"WPI_MotorControlSetOutput.vi"("Output"=0.0, "MotorControlDevRef"=w312) -> ()  [unwired: 7 in, 3 out]
          n122 = call <vilib>:"WPI_MotorControlSetOutput.vi"("Output"=0.0, "MotorControlDevRef"=w314) -> ()  [unwired: 7 in, 3 out]
          n123 = call <vilib>:"WPI_MotorControlSetOutput.vi"("Output"=0.0, "MotorControlDevRef"=w313) -> ()  [unwired: 7 in, 3 out]
        }
        frame #2 {
        }
        frame #3 {
          n124 = call <vilib>:"WPI_SolenoidRefNum Registry Get.vi"("refnum name"="Claw") -> ("error out"=w354:errorcluster, "SolenoidDevRef"=w353:T12)  [unwired: 9 in]
          n125 = call-poly <vilib>:"WPI_SolenoidSet.vi"("error in (no error)"=w354, "Value"=WPI_SolenoidValue."On", "SolenoidDevRef"=w353) -> ("error out"=w357:errorcluster, "SolenoidDevRef"=w358:T12)  [unwired: 7 in]
        }
        frame #4 {
          n126 = Wait (ms)(milliseconds to wait=u32 500) -> ()  [unwired: 1 out]
        }
        frame #5 {
          n127 = call "arm back.vi"() -> ()  [unwired: 12 in]
          n128 = call-poly <vilib>:"WPI_SolenoidSet.vi"("error in (no error)"=w367, "Value"=WPI_SolenoidValue."Off", "SolenoidDevRef"=w368) -> ()  [unwired: 7 in, 2 out]
        }
        frame #6 {
          # "Backs out of community"
          # "+ x is backward in autonomous"
          n129 = while {
            tunnel: [w384] -> w374
            tunnel: [w383] -> w373
            tunnel: w372 -> [w381]
            tunnel: w371 -> [w380]
            tunnel: w370 -> [w378]
            tunnel: w369 -> [w375]
            tunnel: [w375] -> _
            stop <- w382 stop-if-true
            # "198"
            # "makes it drive straight back"
            n130 = call <vilib>:"Spark MAX Get Sensor Position.vi"("MotorControlDevRef in"=w378) -> ("Sensor Position"=w376:dbl)  [unwired: 7 in, 3 out]
            "Sensor Position" <- w376
            n131 = call-poly <vilib>:"WPI_RobotDriveArcadeDrive.vi"("error in (no error)"=w380, "Y axis value"=0.0, "X axis value"=0.7, "RobotDriveDevRef"=w381) -> ("error out"=w383:errorcluster, "RobotDriveDevRef"=w384:T4)  [unwired: 5 in, 1 out]
            n132 = Subtract(x=w376, y=w375) -> (x-y=w377:dbl)
            "Right Drive Encoder" <- w377
            n133 = Greater?(x=w377, y=198.0) -> (0:w382:bool)
          }
          "Timestamp" <- w369
        }
        frame #7 {
          # "Turns 180"
          n134 = while {
            tunnel: w390 -> [w399]
            tunnel: w389 -> [w398]
            tunnel: [w397] -> w388
            tunnel: [w396] -> w387
            stop <- w391 stop-if-true
            n135 = global read "Robot Global Data.vi" "Real Yaw"() -> (w393:dbl)
            "Real Yaw" <- w393
            n136 = call-poly <vilib>:"WPI_RobotDriveArcadeDrive.vi"("error in (no error)"=w398, "Y axis value"=0.4, "X axis value"=0.0, "RobotDriveDevRef"=w399) -> ("error out"=w396:errorcluster, "RobotDriveDevRef"=w397:T4)  [unwired: 5 in, 1 out]
            n137 = In Range and Coerce(upper limit=170.0, x=w393, lower limit=-170.0) -> (In Range?=w392:bool)  [unwired: 1 out]
            n138 = Not(x=w392) -> (.not. x?=w391:bool)
          }
        }
        frame #8 {
          n139 = call-poly <vilib>:"WPI_RobotDriveArcadeDrive.vi"("error in (no error)"=w402, "Y axis value"=0.0, "X axis value"=0.0, "RobotDriveDevRef"=w403) -> ()  [unwired: 5 in, 3 out]
        }
      }
    }
    frame "top cube-balance" {
      n140 = flat-sequence {
        tunnel: w429 -> [w455]
        tunnel: w430 -> [w454]
        tunnel: w431 -> [w453]
        tunnel: [w455] -> w438
        tunnel: [w454] -> w437
        tunnel: [w453] -> w436
        tunnel: w425 -> [w443]
        tunnel: [w439] -> _
        tunnel: w422 -> [w448]
        tunnel: w424 -> [w445]
        tunnel: w423 -> [w439]
        tunnel: w438 -> [w467]
        tunnel: w437 -> [w465]
        tunnel: w436 -> [w466]
        tunnel: [w459] -> w414
        tunnel: [w458] -> w410
        tunnel: [w457] -> w406
        tunnel: [w505] -> w435
        tunnel: [w504] -> w434
        tunnel: [w499] -> w415
        tunnel: w414 -> [w499]
        tunnel: [w498] -> w411
        tunnel: w410 -> [w498]
        tunnel: [w497] -> w407
        tunnel: w406 -> [w497]
        tunnel: w435 -> [w511]
        tunnel: [w511] -> w433
        tunnel: w434 -> [w510]
        tunnel: [w510] -> w432
        tunnel: [w508] -> w416
        tunnel: w415 -> [w508]
        tunnel: [w507] -> w412
        tunnel: w411 -> [w507]
        tunnel: [w506] -> w408
        tunnel: w407 -> [w506]
        tunnel: w433 -> [w517]
        tunnel: w432 -> [w516]
        tunnel: [w514] -> w417
        tunnel: w416 -> [w514]
        tunnel: [w513] -> w413
        tunnel: w412 -> [w513]
        tunnel: [w512] -> w409
        tunnel: w408 -> [w512]
        tunnel: w417 -> [w526]
        tunnel: w413 -> [w525]
        tunnel: w409 -> [w524]
        tunnel: w428 -> [w557]
        tunnel: w427 -> [w556]
        tunnel: [w558] -> w426
        tunnel: [w557] -> w420
        tunnel: [w556] -> w418
        tunnel: w426 -> [w561]
        tunnel: [w560] -> w421
        tunnel: w420 -> [w560]
        tunnel: [w559] -> w419
        tunnel: w418 -> [w559]
        tunnel: w421 -> [w564]
        tunnel: w419 -> [w563]
        frame #0 {
          n141 = Wait (ms)(milliseconds to wait=u32 30) -> ()  [unwired: 1 out]
          n142 = call <vilib>:"Spark MAX Set Sensor Position.vi"("Sensor Type (Hall Sensor)"=Spark_MAX_Sensor_Type."Hall Sensor", "Position"=0.0, "MotorControlDeviceRef"=w443) -> ("MotorControlDeviceRef"=w442:T5)  [unwired: 7 in, 1 out]
          n143 = call <vilib>:"Spark MAX Set Sensor Position.vi"("Sensor Type (Hall Sensor)"=Spark_MAX_Sensor_Type."Hall Sensor", "Position"=0.0, "MotorControlDeviceRef"=w445) -> ()  [unwired: 7 in, 2 out]
          n144 = call <vilib>:"Spark MAX Get Sensor Position.vi"("MotorControlDevRef in"=w442) -> ()  [unwired: 7 in, 4 out]
          n145 = call <vilib>:"Spark MAX Set Sensor Position.vi"("Sensor Type (Hall Sensor)"=Spark_MAX_Sensor_Type."Hall Sensor", "Position"=0.0, "MotorControlDeviceRef"=w448) -> ()  [unwired: 7 in, 2 out]
          n146 = call <vilib>:"Spark MAX Set Sensor Position.vi"("Sensor Type (Hall Sensor)"=Spark_MAX_Sensor_Type."Hall Sensor", "Position"=0.0, "MotorControlDeviceRef"=w439) -> ()  [unwired: 7 in, 2 out]
        }
        frame #1 {
          n147 = while {
            tunnel: w466 -> [w473]
            tunnel: w465 -> [w472]
            tunnel: w467 -> [w471]
            tunnel: [w468] -> w456
            tunnel: [w470] -> w464
            tunnel: [w469] -> w463
            stop <- w496 stop-if-true
            n148 = global read "Robot Global Data.vi" "Arm Blue"() -> (w476:dbl)
            n149 = global read "Robot Global Data.vi" "Arm Red"() -> (w487:dbl)
            n150 = Subtract(x=145.592, y=w487) -> (x-y=w474:dbl)
            n151 = Subtract(x=67.2, y=w476) -> (x-y=w475:dbl)
            n152 = Multiply(x=w475, y=0.5) -> (x*y=w484:dbl)
            n153 = Multiply(x=w474, y=-0.5) -> (x*y=w483:dbl)
            n154 = In Range and Coerce(upper limit=1.0, x=w475, lower limit=-1.0) -> (In Range?=w495:bool)  [unwired: 1 out]
            n155 = In Range and Coerce(upper limit=1.0, x=w474, lower limit=-1.0) -> (In Range?=w494:bool)  [unwired: 1 out]
            n156 = In Range and Coerce(upper limit=0.2, x=w484, lower limit=-0.2) -> (coerced(x)=w479:dbl)  [unwired: 1 out]
            n157 = In Range and Coerce(upper limit=0.6, x=w483, lower limit=-0.6) -> (coerced(x)=w480:dbl)  [unwired: 1 out]
            n158 = call <vilib>:"WPI_MotorControlSetOutput.vi"("Output"=w479, "MotorControlDevRef"=w472) -> ("MotorControlDevRef"=w468:T5)  [unwired: 7 in, 2 out]
            n159 = call <vilib>:"WPI_MotorControlSetOutput.vi"("Output"=w479, "MotorControlDevRef"=w471) -> ("MotorControlDevRef"=w470:T5)  [unwired: 7 in, 2 out]
            n160 = call <vilib>:"WPI_MotorControlSetOutput.vi"("Output"=w480, "MotorControlDevRef"=w473) -> ("MotorControlDevRef"=w469:T5)  [unwired: 7 in, 2 out]
            n161 = And(x=w495, y=w494) -> (x .and. y?=w496:bool)
          }
          n162 = call <vilib>:"WPI_MotorControlSetOutput.vi"("Output"=0.0, "MotorControlDevRef"=w463) -> ("MotorControlDevRef"=w459:T5)  [unwired: 7 in, 2 out]
          n163 = call <vilib>:"WPI_MotorControlSetOutput.vi"("Output"=0.0, "MotorControlDevRef"=w456) -> ("MotorControlDevRef"=w458:T5)  [unwired: 7 in, 2 out]
          n164 = call <vilib>:"WPI_MotorControlSetOutput.vi"("Output"=0.0, "MotorControlDevRef"=w464) -> ("MotorControlDevRef"=w457:T5)  [unwired: 7 in, 2 out]
        }
        frame #2 {
          n165 = call <vilib>:"WPI_SolenoidRefNum Registry Get.vi"("refnum name"="Claw") -> ("error out"=w503:errorcluster, "SolenoidDevRef"=w502:T12)  [unwired: 9 in]
          n166 = call-poly <vilib>:"WPI_SolenoidSet.vi"("error in (no error)"=w503, "Value"=WPI_SolenoidValue."On", "SolenoidDevRef"=w502) -> ("error out"=w504:errorcluster, "SolenoidDevRef"=w505:T12)  [unwired: 7 in]
        }
        frame #3 {
          n167 = Wait (ms)(milliseconds to wait=u32 500) -> ()  [unwired: 1 out]
        }
        frame #4 {
          n168 = call-poly <vilib>:"WPI_SolenoidSet.vi"("error in (no error)"=w516, "Value"=WPI_SolenoidValue."Off", "SolenoidDevRef"=w517) -> ()  [unwired: 7 in, 2 out]
        }
        frame #5 {
          # "puts arm in"
          n169 = while {
            tunnel: w526 -> [w532]
            tunnel: w525 -> [w531]
            tunnel: w524 -> [w527]
            tunnel: [w528] -> w523
            tunnel: [w530] -> w522
            tunnel: [w529] -> w521
            stop <- w555 stop-if-true
            n170 = global read "Robot Global Data.vi" "Arm Blue"() -> (w535:dbl)
            n171 = global read "Robot Global Data.vi" "Arm Red"() -> (w546:dbl)
            n172 = Subtract(x=20.0, y=w546) -> (x-y=w533:dbl)
            n173 = Subtract(x=0.0, y=w535) -> (x-y=w534:dbl)
            n174 = Multiply(x=w534, y=0.5) -> (x*y=w543:dbl)
            n175 = Multiply(x=w533, y=-0.5) -> (x*y=w542:dbl)
            n176 = In Range and Coerce(upper limit=1.0, x=w534, lower limit=-1.0) -> (In Range?=w554:bool)  [unwired: 1 out]
            n177 = In Range and Coerce(upper limit=1.0, x=w533, lower limit=-1.0) -> (In Range?=w553:bool)  [unwired: 1 out]
            n178 = In Range and Coerce(upper limit=0.6, x=w543, lower limit=-0.6) -> (coerced(x)=w538:dbl)  [unwired: 1 out]
            n179 = In Range and Coerce(upper limit=0.5, x=w542, lower limit=-0.5) -> (coerced(x)=w539:dbl)  [unwired: 1 out]
            n180 = call <vilib>:"WPI_MotorControlSetOutput.vi"("Output"=w538, "MotorControlDevRef"=w531) -> ("MotorControlDevRef"=w528:T5)  [unwired: 7 in, 2 out]
            n181 = call <vilib>:"WPI_MotorControlSetOutput.vi"("Output"=w538, "MotorControlDevRef"=w527) -> ("MotorControlDevRef"=w530:T5)  [unwired: 7 in, 2 out]
            n182 = call <vilib>:"WPI_MotorControlSetOutput.vi"("Output"=w539, "MotorControlDevRef"=w532) -> ("MotorControlDevRef"=w529:T5)  [unwired: 7 in, 2 out]
            n183 = And(x=w554, y=w553) -> (x .and. y?=w555:bool)
          }
          n184 = call <vilib>:"WPI_MotorControlSetOutput.vi"("Output"=0.0, "MotorControlDevRef"=w521) -> ()  [unwired: 7 in, 3 out]
          n185 = call <vilib>:"WPI_MotorControlSetOutput.vi"("Output"=0.0, "MotorControlDevRef"=w523) -> ()  [unwired: 7 in, 3 out]
          n186 = call <vilib>:"WPI_MotorControlSetOutput.vi"("Output"=0.0, "MotorControlDevRef"=w522) -> ()  [unwired: 7 in, 3 out]
        }
        frame #6 {
          n187 = Tick Count (ms)() -> (millisecond timer value=w558:u32)
        }
        frame #7 {
          n188 = call "Balance.vi"("Start Time"=w561, "Boolean"=TRUE) -> ()  [unwired: 10 in]
        }
        frame #8 {
          n189 = call-poly <vilib>:"WPI_RobotDriveArcadeDrive.vi"("error in (no error)"=w563, "Y axis value"=0.0, "X axis value"=0.0, "RobotDriveDevRef"=w564) -> ()  [unwired: 5 in, 3 out]
        }
      }
    }
    frame "top cube" {
      n190 = flat-sequence {
        tunnel: w590 -> [w611]
        tunnel: w591 -> [w610]
        tunnel: w592 -> [w609]
        tunnel: [w611] -> w585
        tunnel: [w599] -> w580
        tunnel: [w610] -> w579
        tunnel: [w609] -> w578
        tunnel: w577 -> [w596]
        tunnel: w576 -> [w606]
        tunnel: w575 -> [w603]
        tunnel: w574 -> [w600]
        tunnel: [w598] -> w569
        tunnel: w585 -> [w622]
        tunnel: [w621] -> w581
        tunnel: w580 -> [w621]
        tunnel: w579 -> [w619]
        tunnel: w578 -> [w620]
        tunnel: [w618] -> w570
        tunnel: w569 -> [w618]
        tunnel: [w653] -> w582
        tunnel: w581 -> [w653]
        tunnel: [w652] -> w571
        tunnel: w570 -> [w652]
        tunnel: [w661] -> w589
        tunnel: [w660] -> w587
        tunnel: [w659] -> w583
        tunnel: w582 -> [w659]
        tunnel: [w658] -> w572
        tunnel: w571 -> [w658]
        tunnel: w589 -> [w666]
        tunnel: [w666] -> w588
        tunnel: w587 -> [w665]
        tunnel: [w665] -> w586
        tunnel: [w664] -> w584
        tunnel: w583 -> [w664]
        tunnel: [w663] -> w573
        tunnel: w572 -> [w663]
        tunnel: w588 -> [w670]
        tunnel: w586 -> [w669]
        tunnel: w584 -> [_]
        tunnel: w573 -> [_]
        tunnel: [w668] -> w568
        tunnel: w567 -> [w668]
        tunnel: w568 -> [w671]
        frame #0 {
          n191 = Wait (ms)(milliseconds to wait=u32 30) -> ()  [unwired: 1 out]
          n192 = call <vilib>:"Spark MAX Set Sensor Position.vi"("Sensor Type (Hall Sensor)"=Spark_MAX_Sensor_Type."Hall Sensor", "Position"=0.0, "MotorControlDeviceRef"=w596) -> ("MotorControlDeviceRef"=w595:T5)  [unwired: 7 in, 1 out]
          n193 = call <vilib>:"Spark MAX Set Sensor Position.vi"("Sensor Type (Hall Sensor)"=Spark_MAX_Sensor_Type."Hall Sensor", "Position"=0.0, "MotorControlDeviceRef"=w600) -> ()  [unwired: 7 in, 2 out]
          n194 = call <vilib>:"Spark MAX Get Sensor Position.vi"("MotorControlDevRef in"=w595) -> ("Sensor Position"=w598:dbl, "MotorControlDevRef out"=w599:T5)  [unwired: 7 in, 2 out]
          n195 = call <vilib>:"Spark MAX Set Sensor Position.vi"("Sensor Type (Hall Sensor)"=Spark_MAX_Sensor_Type."Hall Sensor", "Position"=0.0, "MotorControlDeviceRef"=w603) -> ()  [unwired: 7 in, 2 out]
          n196 = call <vilib>:"Spark MAX Set Sensor Position.vi"("Sensor Type (Hall Sensor)"=Spark_MAX_Sensor_Type."Hall Sensor", "Position"=0.0, "MotorControlDeviceRef"=w606) -> ()  [unwired: 7 in, 2 out]
        }
        frame #1 {
          n197 = while {
            tunnel: w620 -> [w628]
            tunnel: w619 -> [w627]
            tunnel: w622 -> [w626]
            tunnel: [w623] -> w617
            tunnel: [w625] -> w616
            tunnel: [w624] -> w615
            stop <- w651 stop-if-true
            n198 = global read "Robot Global Data.vi" "Arm Blue"() -> (w631:dbl)
            n199 = global read "Robot Global Data.vi" "Arm Red"() -> (w642:dbl)
            n200 = Subtract(x=145.592, y=w642) -> (x-y=w629:dbl)
            n201 = Subtract(x=67.2, y=w631) -> (x-y=w630:dbl)
            n202 = Multiply(x=w630, y=0.5) -> (x*y=w639:dbl)
            n203 = Multiply(x=w629, y=-0.5) -> (x*y=w638:dbl)
            n204 = In Range and Coerce(upper limit=1.0, x=w630, lower limit=-1.0) -> (In Range?=w650:bool)  [unwired: 1 out]
            n205 = In Range and Coerce(upper limit=1.0, x=w629, lower limit=-1.0) -> (In Range?=w649:bool)  [unwired: 1 out]
            n206 = In Range and Coerce(upper limit=0.2, x=w639, lower limit=-0.2) -> (coerced(x)=w634:dbl)  [unwired: 1 out]
            n207 = In Range and Coerce(upper limit=0.6, x=w638, lower limit=-0.6) -> (coerced(x)=w635:dbl)  [unwired: 1 out]
            n208 = call <vilib>:"WPI_MotorControlSetOutput.vi"("Output"=w634, "MotorControlDevRef"=w627) -> ("MotorControlDevRef"=w623:T5)  [unwired: 7 in, 2 out]
            n209 = call <vilib>:"WPI_MotorControlSetOutput.vi"("Output"=w634, "MotorControlDevRef"=w626) -> ("MotorControlDevRef"=w625:T5)  [unwired: 7 in, 2 out]
            n210 = call <vilib>:"WPI_MotorControlSetOutput.vi"("Output"=w635, "MotorControlDevRef"=w628) -> ("MotorControlDevRef"=w624:T5)  [unwired: 7 in, 2 out]
            n211 = And(x=w650, y=w649) -> (x .and. y?=w651:bool)
          }
          n212 = call <vilib>:"WPI_MotorControlSetOutput.vi"("Output"=0.0, "MotorControlDevRef"=w615) -> ()  [unwired: 7 in, 3 out]
          n213 = call <vilib>:"WPI_MotorControlSetOutput.vi"("Output"=0.0, "MotorControlDevRef"=w617) -> ()  [unwired: 7 in, 3 out]
          n214 = call <vilib>:"WPI_MotorControlSetOutput.vi"("Output"=0.0, "MotorControlDevRef"=w616) -> ()  [unwired: 7 in, 3 out]
        }
        frame #2 {
        }
        frame #3 {
          n215 = call <vilib>:"WPI_SolenoidRefNum Registry Get.vi"("refnum name"="Claw") -> ("error out"=w657:errorcluster, "SolenoidDevRef"=w656:T12)  [unwired: 9 in]
          n216 = call-poly <vilib>:"WPI_SolenoidSet.vi"("error in (no error)"=w657, "Value"=WPI_SolenoidValue."On", "SolenoidDevRef"=w656) -> ("error out"=w660:errorcluster, "SolenoidDevRef"=w661:T12)  [unwired: 7 in]
        }
        frame #4 {
          n217 = Wait (ms)(milliseconds to wait=u32 500) -> ()  [unwired: 1 out]
        }
        frame #5 {
          n218 = call-poly <vilib>:"WPI_SolenoidSet.vi"("error in (no error)"=w669, "Value"=WPI_SolenoidValue."Off", "SolenoidDevRef"=w670) -> ()  [unwired: 7 in, 2 out]
        }
        frame #6 {
          n219 = call-poly <vilib>:"WPI_RobotDriveArcadeDrive.vi"("Y axis value"=0.0, "X axis value"=0.0, "RobotDriveDevRef"=w671) -> ()  [unwired: 6 in, 3 out]
        }
      }
    }
    frame "Balance" {
      # "You can put your main auto here, or you can right-click on the case and make any\nother frame be the default case."
      # "This is the frame that will execute if no selection is made, or if it is not recognized"
      n220 = flat-sequence {
        tunnel: [w675] -> w674
        tunnel: w674 -> [w677]
        frame #0 {
          n221 = Tick Count (ms)() -> (millisecond timer value=w675:u32)
        }
        frame #1 {
          n222 = call "Balance.vi"("Start Time"=w677, "Boolean"=TRUE) -> ()  [unwired: 10 in]
        }
      }
    }
    frame "Drive Straight" {
      n223 = flat-sequence {
        tunnel: [w683] -> w680
        tunnel: w679 -> [w683]
        tunnel: [w689] -> w682
        tunnel: [w688] -> w681
        tunnel: w680 -> [w686]
        tunnel: w678 -> [w685]
        tunnel: w682 -> [w702]
        tunnel: w681 -> [w701]
        frame #0 {
          # "Creates the starting angle"
          n224 = global read "Robot Global Data.vi" "yaw"() -> (w684:dbl)
          n225 = global write "Robot Global Data.vi" "Gyro Starting Value in our match"(w684) -> ()
        }
        frame #1 {
          n226 = Tick Count (ms)() -> (millisecond timer value=w687:u32)
          n227 = while {
            tunnel: [w699] -> w689
            tunnel: [w698] -> w688
            tunnel: w687 -> [w696]
            tunnel: w686 -> [w691]
            tunnel: w685 -> [w690]
            stop <- w692 stop-if-true
            n228 = call "Drive straight.vi"("Start Time"=w696, "Length(seconds)"=6.0, "Desired angle"=0.0) -> ("Complete or not"=w692:bool, "X Power"=w693:dbl)  [unwired: 7 in]
            n229 = Wait (ms)(milliseconds to wait=u32 10) -> ()  [unwired: 1 out]
            n230 = call-poly <vilib>:"WPI_RobotDriveArcadeDrive.vi"("error in (no error)"=w690, "Y axis value"=-0.55, "X axis value"=w693, "RobotDriveDevRef"=w691) -> ("error out"=w698:errorcluster, "RobotDriveDevRef"=w699:T4)  [unwired: 5 in, 1 out]
          }
        }
        frame #2 {
          n231 = call-poly <vilib>:"WPI_RobotDriveArcadeDrive.vi"("error in (no error)"=w701, "Y axis value"=0.0, "X axis value"=0.0, "RobotDriveDevRef"=w702) -> ()  [unwired: 5 in, 3 out]
        }
      }
    }
    frame "Test Balance" {
      n232 = flat-sequence {
        tunnel: w708 -> [w712]
        tunnel: w707 -> [w711]
        tunnel: [w710] -> w706
        tunnel: [w709] -> w705
        tunnel: w706 -> [w725]
        tunnel: w705 -> [w724]
        frame #0 {
          n233 = while {
            shift-right: [w718] -> w709
            shift-left: w712 -> [w721]
            shift-right: [w719] -> w710
            shift-left: w711 -> [w720]
            stop <- w713 stop-if-true
            n234 = global read "Robot Global Data.vi" "Pitch"() -> (w715:dbl)
            n235 = call-poly <vilib>:"WPI_RobotDriveArcadeDrive.vi"("error in (no error)"=w720, "Y axis value"=-0.55, "X axis value"=0.0, "RobotDriveDevRef"=w721) -> ("error out"=w719:errorcluster, "RobotDriveDevRef"=w718:T4)  [unwired: 5 in, 1 out]
            n236 = In Range and Coerce(upper limit=10.0, x=w715, lower limit=-10.0 ("y")) -> (In Range?=w716:bool)  [unwired: 1 out]
            n237 = Not(x=w716) -> (.not. x?=w713:bool)
          }
        }
        frame #1 {
          n238 = while {
            tunnel: w725 -> [w727]
            tunnel: w724 -> [w726]
            stop <- FALSE stop-if-true
            n239 = call "Derivative balance.vi"() -> ("Motor Power"=w730:dbl)  [unwired: 11 in]
            n240 = call-poly <vilib>:"WPI_RobotDriveArcadeDrive.vi"("error in (no error)"=w727, "Y axis value"=w730, "X axis value"=0.0, "RobotDriveDevRef"=w726) -> ()  [unwired: 5 in, 3 out]
          }
        }
      }
    }
    frame Default {
    }
  }
